vi "Launch.vi"() -> ()   [LabVIEW 2019]
uses:
  Components/ViPER.lvlibp/1abvi3w/ProjectTemplates/Source/Core/ViPER/Components_Src/ViPER/ViPER.lvclass
panel:
  out "error out":errorcluster
  in  "Config XML":string="        <Object>\n          <Name>DMM</Name>\n          <Class>DMM_Keysight_34980A</Class>\n          <Config>\n            <NumElts>1</NumElts>\n            <Refnum>\n              <Name>VISA</Name>\n              <RefKind>VISA</RefKind>\n              <Val>USB0::0x0957::0x0507::MY56485422::INSTR</Val>\n</Refnum>\n</Config>        </Object>"
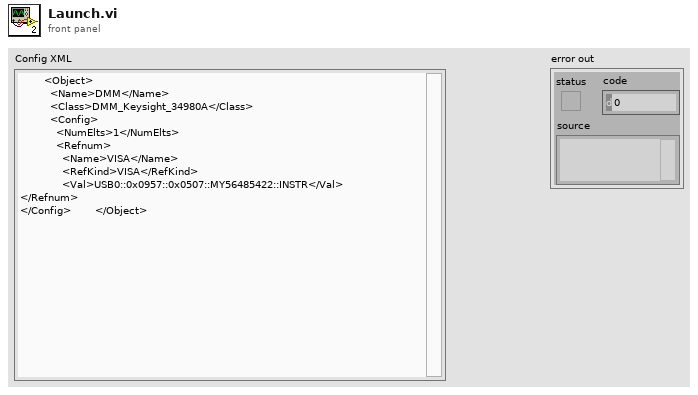
[diagram p1: front panel]
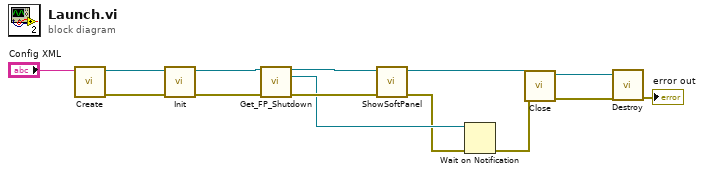
[diagram p0: block diagram]
diagram:
  n1 = call "Create.vi"("Config XML"="Config XML") -> ("error out"=w13:errorcluster, "reference out"=w14:refnum<class "ViPER.lvclass">)  [unwired: 9 in]
  n2 = call-dynamic "Init.vi"("error in (no error)"=w13, "reference in"=w14) -> ("error out"=w11:errorcluster, "reference out"=w12:refnum<class "ViPER.lvclass">)  [unwired: 8 in]
  n3 = call "Get_FP_Shutdown.vi"("ViPER_Base in"=w12, "error in (no error)"=w11) -> ("ViPER_Base out"=w10:refnum<class "ViPER.lvclass">, "SoftFP_Shutdown"=w8:refnum<notifier>, "error out"=w9:errorcluster)  [unwired: 9 in, 2 out]
  n4 = call-dynamic "ShowSoftPanel.vi"("error in (no error)"=w9, "Driver in"=w10) -> ("error out"=w7:errorcluster, "Driver out"=w6:refnum<class "ViPER.lvclass">)  [unwired: 7 in, 1 out]
  n5 = Wait on Notification(notifier=w8, error in (no error)=w7) -> (error out=w5:errorcluster)  [unwired: 2 in, 3 out]
  n6 = call-dynamic "Close.vi"("error in (no error)"=w5, "reference in"=w6) -> ("error out"=w4:errorcluster, "reference out"=w3:refnum<class "ViPER.lvclass">)  [unwired: 8 in]
  n7 = call "Destroy.vi"("error in (no error)"=w4, "reference in"=w3) -> ("error out"=→"error out":errorcluster)  [unwired: 9 in]
